vi "Assign Shared Resource.vi"(8 "error in (no error)":errorcluster, 10 "UUID":string, 11 "Controller in":refnum<class "Controller.lvclass">) -> (0 "error out":errorcluster, 3 "Controller out":refnum<class "Controller.lvclass">)   [LabVIEW 2013, in "SET Project Editor.lvlib" / "Controller.lvclass"]
uses:
  Controller.lvclass
  Controller.lvclass/Controller.ctl
  SET Project Data/Project Data Class/Project Data.lvclass
  SET Project Data/VI Class/VI Data.lvclass
  SET Project Data/Control Classes/GObject/GObject.lvclass/GObject.ctl
  <vilib>/ActorFramework/Message Enqueuer/Message Enqueuer.lvclass/Message Enqueuer.ctl
  SET Project Data/Menu Class/Menu Data.lvclass/Menu Data.ctl
  SET Project Data/Control Classes/GObject/Read Items.vi
  SET Project Data/Control Classes/GObject/Write Items.vi
  SET Project Data/Menu Class/Read Menu Item LUT.vi
  SET Project Data/Menu Class/Write Menu Item LUT.vi
  <vilib>/ActorFramework/Message Enqueuer/Enqueue.vi
  <vilib>/ActorFramework/Message Priority Queue/Priority Enqueue.vi
  SET Project Data/Resource Data Class/Resource Data.lvclass
  UI View Messages/UI Refresh Data Msg/UI Refresh Data Msg.lvclass
  SET Project Editor.lvlib
  SET Project Data/Control Classes/GObject/GObject.lvclass
  SET Project Data/Menu Class/Menu Data.lvclass
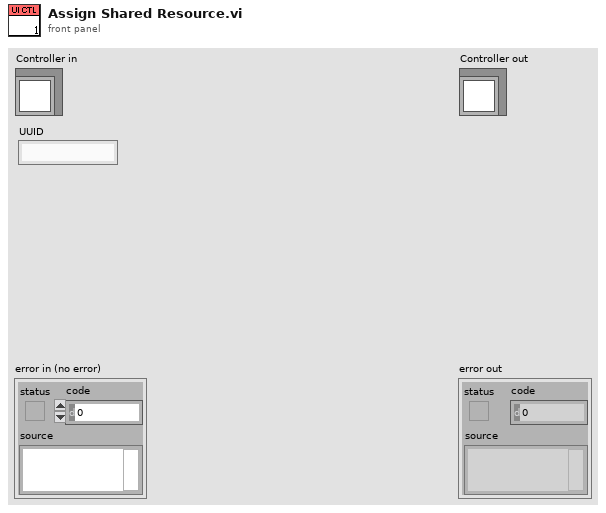
[diagram p1: front panel]
types:
  T1 = typedef "SET Project Editor.lvlib/UID Types.ctl" = enum16{"Invalid", "VI File", "GObject", "GObject Item", "RTM File", "RTM Item"}
  T2 = typedef "SET Project Data.lvlib/ProjFile_Resource Entry.ctl" = cluster{"RID":string, "Tag":string, "Strings [] (UTF-16)":string[], "Shared?":bool}
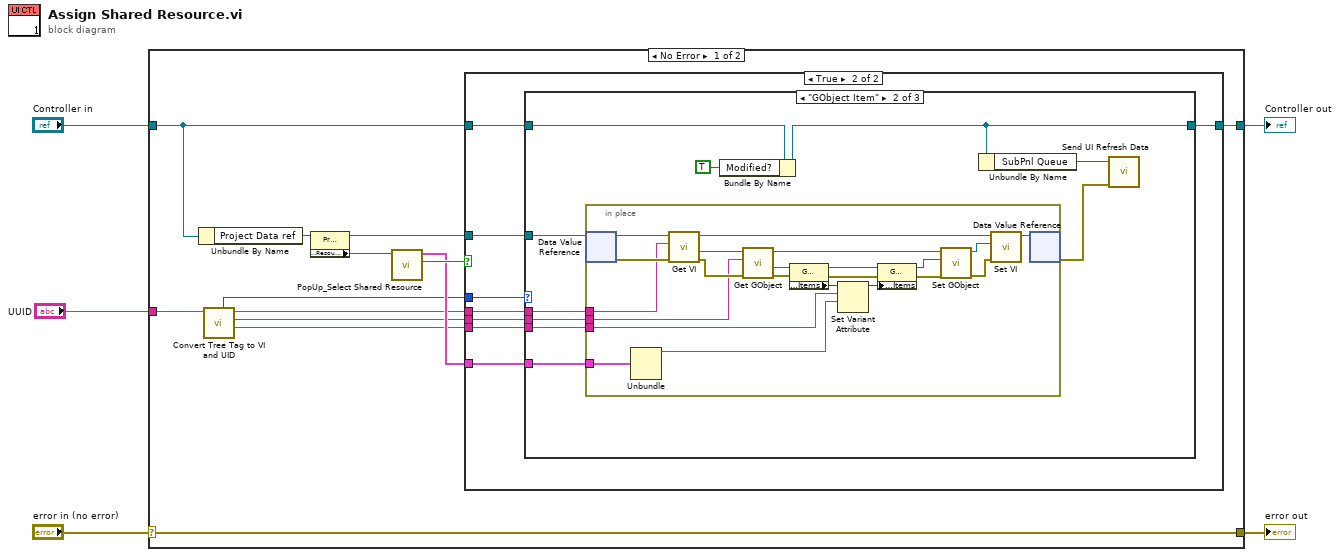
[diagram p0: block diagram]
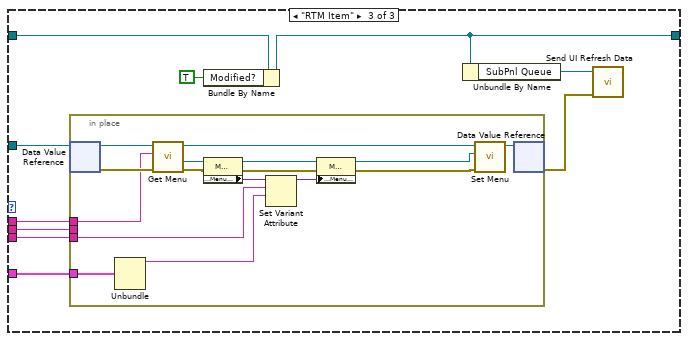
[diagram p4: hidden frame]
diagram:
  n1 = case shown="No Error" "error in (no error)" {
    selector: "error in (no error)" -> [w18 w88]
    tunnel: [w18 w88] -> w4
    tunnel: [w11 w87] -> w2
    tunnel: "Controller in" -> [w12 w87]
    tunnel: "UUID" -> [w10 _]
    frame No Error {
      n2 = Unbundle By Name(w12) -> ("Project Data ref"=w17:refnum<data-value>)
      n3 = call "Convert Tree Tag to VI and UID.vi"("Tree Tag"=w10) -> ("Item Name"=w7:string, "GObject UID"=w8:string, "File Path (Relative)"=w9:string, "UID Type"=w6:T1)  [unwired: 7 in]
      n4 = property class="Project Data.lvclass"(reference=w17) -> (reference out=w16:refnum<data-value>, "Properties:Resource Data ref"=w15:refnum<data-value>)  [unwired: 1 in, 1 out]
      n5 = call "PopUp_Select Shared Resource.vi"("*ResData"=w15) -> ("OK Pressed?"=w14:bool, "Resource"=w13:T2)  [unwired: 8 in, 1 out]
      n6 = case shown="True" w14 {
        tunnel: w16 -> [_ w27]
        tunnel: w13 -> [_ w26]
        tunnel: w12 -> [w19 w25]
        tunnel: [w19 w24] -> w11
        tunnel: w9 -> [_ w23]
        tunnel: w8 -> [_ w22]
        tunnel: w7 -> [_ w21]
        tunnel: w6 -> [_ w20]
        frame False {
        }
        frame True {
          n7 = case shown="\"GObject Item\"" w20 {
            tunnel: w27 -> [_ w38 w70]
            tunnel: w26 -> [_ w37 w69]
            tunnel: w25 -> [w28 w35 w67]
            tunnel: [w28 w34 w66] -> w24
            tunnel: w23 -> [_ w32 w64]
            tunnel: w22 -> [_ w31 w63]
            tunnel: w21 -> [_ w30 w62]
            frame "Invalid", Default {
              # "#TODO - Warning or error"
              # "Should not be here..."
            }
            frame "GObject Item" {
              n8 = in-place {
                in-place-border: w37 -> [w46]
                in-place-border: w32 -> [w44]
                in-place-border: w31 -> [w43]
                in-place-border: w30 -> [w42]
                n9 = in-place-dvr #1(w38) -> (w60:refnum<class "Project Data.lvclass">, w57:errorcluster)
                n10 = Unbundle(w46) -> ("RID"=w45:string)  [unwired: 3 out]
                n11 = call-dynamic "Get VI.vi"("error in (no error)"=w57, "VI Path (Relative)"=w44, "ProjectData in"=w60) -> ("error out"=w58:errorcluster, "VI Data out"=w59:refnum<class "VI Data.lvclass">, "ProjectData out"=w55:refnum<class "Project Data.lvclass">)  [unwired: 5 in, 1 out]
                n12 = call-dynamic "Get GObject.vi"("error in (no error)"=w58, "GObject UID"=w43, "VI Data in"=w59) -> ("error out"=w41:errorcluster, "GObject"=w52:refnum<class "GObject.lvclass">, "VI Data out"=w56:refnum<class "VI Data.lvclass">)  [unwired: 5 in, 1 out]
                n13 = property class="GObject.lvclass"(reference=w52, error in=w41) -> (reference out=w47:refnum<class "GObject.lvclass">, error out=w40:errorcluster, "Properties:Items"=w49:variant)
                n14 = Set Variant Attribute(Variant=w49, name=w42, value=w45) -> (Variant out=w48:variant)  [unwired: 1 in, 2 out]
                n15 = property class="GObject.lvclass"(reference=w47, error in=w40, "Properties:Items"=w48) -> (reference out=w51:refnum<class "GObject.lvclass">, error out=w50:errorcluster)
                n16 = call "Set GObject.vi"("error in (no error)"=w50, "GObject.lvclass"=w51, "VI Data in"=w56) -> ("error out"=w39:errorcluster, "VI Data out"=w54:refnum<class "VI Data.lvclass">)  [unwired: 6 in, 1 out]
                n17 = call-dynamic "Set VI.vi"("error in (no error)"=w39, "VI Data in"=w54, "ProjectData in"=w55) -> ("ProjectData out"=w53:refnum<class "Project Data.lvclass">)  [unwired: 6 in, 2 out]
                n18 = in-place-dvr #1(w53) -> (w29:errorcluster)  [unwired: 1 out]
              }
              n19 = Bundle By Name(cluster=w35, "Modified?"=TRUE) -> (w34:refnum<class "Controller.lvclass">)
              n20 = Unbundle By Name(w34) -> ("SubPnl Queue"=w36:refnum<class "Message Enqueuer.lvclass">)
              n21 = call "Send UI Refresh Data.vi"("error in (no error)"=w29, "Message Enqueuer"=w36) -> ()  [unwired: 8 in, 2 out]
            }
            frame "RTM Item" {
              n22 = in-place {
                in-place-border: w69 -> [w82]
                in-place-border: w64 -> [w80]
                in-place-border: w63 -> [_]
                in-place-border: w62 -> [w79]
                n23 = in-place-dvr #2(w70) -> (w86:refnum<class "Project Data.lvclass">, w85:errorcluster)
                n24 = Unbundle(w82) -> ("RID"=w81:string)  [unwired: 3 out]
                n25 = call-dynamic "Get Menu.vi"("error in (no error)"=w85, "Menu Path (Relative)"=w80, "ProjectData in"=w86) -> ("error out"=w73:errorcluster, "Menu Data out"=w78:refnum<class "Menu Data.lvclass">, "ProjectData out"=w84:refnum<class "Project Data.lvclass">)  [unwired: 5 in, 1 out]
                n26 = property class="Menu Data.lvclass"(reference=w78, error in=w73) -> (reference out=w76:refnum<class "Menu Data.lvclass">, error out=w72:errorcluster, "Properties:Menu Item LUT"=w77:variant)
                n27 = Set Variant Attribute(Variant=w77, name=w79, value=w81) -> (Variant out=w75:variant)  [unwired: 1 in, 2 out]
                n28 = property class="Menu Data.lvclass"(reference=w76, error in=w72, "Properties:Menu Item LUT"=w75) -> (reference out=w74:refnum<class "Menu Data.lvclass">, error out=w71:errorcluster)
                n29 = call-dynamic "Set Menu.vi"("error in (no error)"=w71, "RTM Data in"=w74, "ProjectData in"=w84) -> ("ProjectData out"=w83:refnum<class "Project Data.lvclass">)  [unwired: 6 in, 2 out]
                n30 = in-place-dvr #2(w83) -> (w61:errorcluster)  [unwired: 1 out]
              }
              n31 = Bundle By Name(cluster=w67, "Modified?"=TRUE) -> (w66:refnum<class "Controller.lvclass">)
              n32 = Unbundle By Name(w66) -> ("SubPnl Queue"=w68:refnum<class "Message Enqueuer.lvclass">)
              n33 = call "Send UI Refresh Data.vi"("error in (no error)"=w61, "Message Enqueuer"=w68) -> ()  [unwired: 8 in, 2 out]
            }
          }
        }
      }
    }
    frame Error {
    }
  }
  "error out" <- w4
  "Controller out" <- w2
